vi "Saving_Data.vi"(5 "Current":dbl, 7 "Watt":dbl, 8 "Voltage":dbl, 9 "RPM":dbl, 10 "Iteration":i32, 11 "file path":path) -> ()   [LabVIEW 2023, in "Test_Libraries.lvlib"]
uses:
  Proyecto/Test_Libraries.lvlib
  <vilib>/Utility/file.llb/Write Delimited Spreadsheet (string).vi
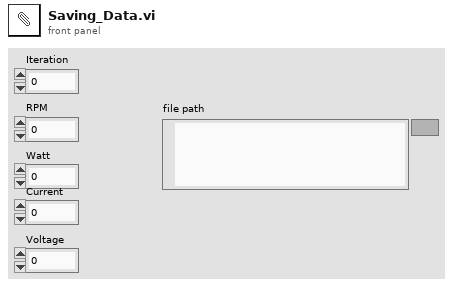
[diagram p1: front panel]
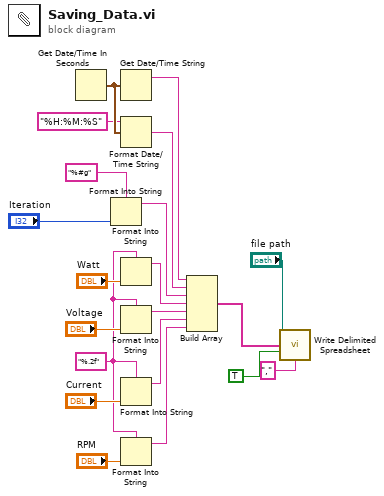
[diagram p0: block diagram]
diagram:
  w6 = "%.2f" ("format string")
  n1 = Get Date/Time In Seconds() -> (seconds since 1Jan1904=w18:timestamp)
  n2 = Format Into String(format string="%#g", "Iteration") -> (resulting string=w13:string)  [unwired: 2 in, 1 out]
  n3 = Get Date/Time String(seconds (now)=w18) -> (date string=w19:string)  [unwired: 2 in, 1 out]
  n4 = Format Date/Time String(time format string (%c)="%H:%M:%S", seconds (now)=w18) -> (date/time string=w20:string)  [unwired: 1 in]
  n5 = Format Into String(format string=w6, "Watt") -> (resulting string=w14:string)  [unwired: 2 in, 1 out]
  n6 = Format Into String(format string=w6, "Voltage") -> (resulting string=w15:string)  [unwired: 2 in, 1 out]
  n7 = Format Into String(format string=w6, "Current") -> (resulting string=w16:string)  [unwired: 2 in, 1 out]
  n8 = Format Into String(format string=w6, "RPM") -> (resulting string=w17:string)  [unwired: 2 in, 1 out]
  n9 = Build Array(w19, w20, w13, w14, w15, w16, w17) -> (w2:string[])
  n10 = call-poly <vilib>:"Write Delimited Spreadsheet.vi"("file path (dialog if empty)"="file path", "1D data"=w2, "append to file? (new file:F)"=TRUE, "delimiter (\\t)"="," ("delimiter (\\t)")) -> ()  [unwired: 10 in, 2 out]
